vi "Roborealm image string.vi"(4 "remote port or service name":u16=1180, 6 "UP IP Address":string, 7 "Camera":string, 8 "error in (no error)":errorcluster, 9 "Width":string, 10 "Height":string, 11 "TCP Network Connection in":refnum<k5>) -> (0 "error out":errorcluster, 2 "connection ID out":refnum<k5>, 3 "String":string)   [LabVIEW 2017]
panel:
  out "img":string
  out "output 3":u32
  out "output 2":u32
  out "output 1":u32
  out "offset past scan":u32
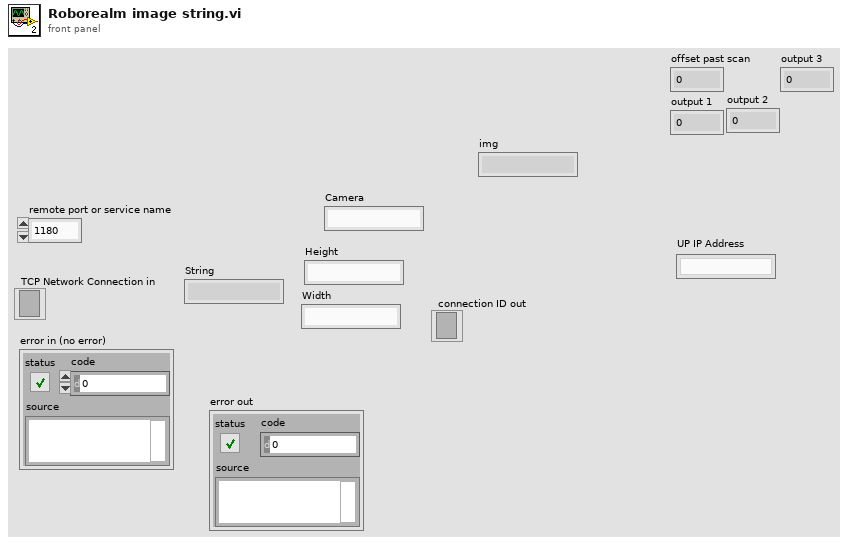
[diagram p1: front panel]
types:
  T1 = enum16{"Standard", "Buffered", "CRLF", "Immediate"}
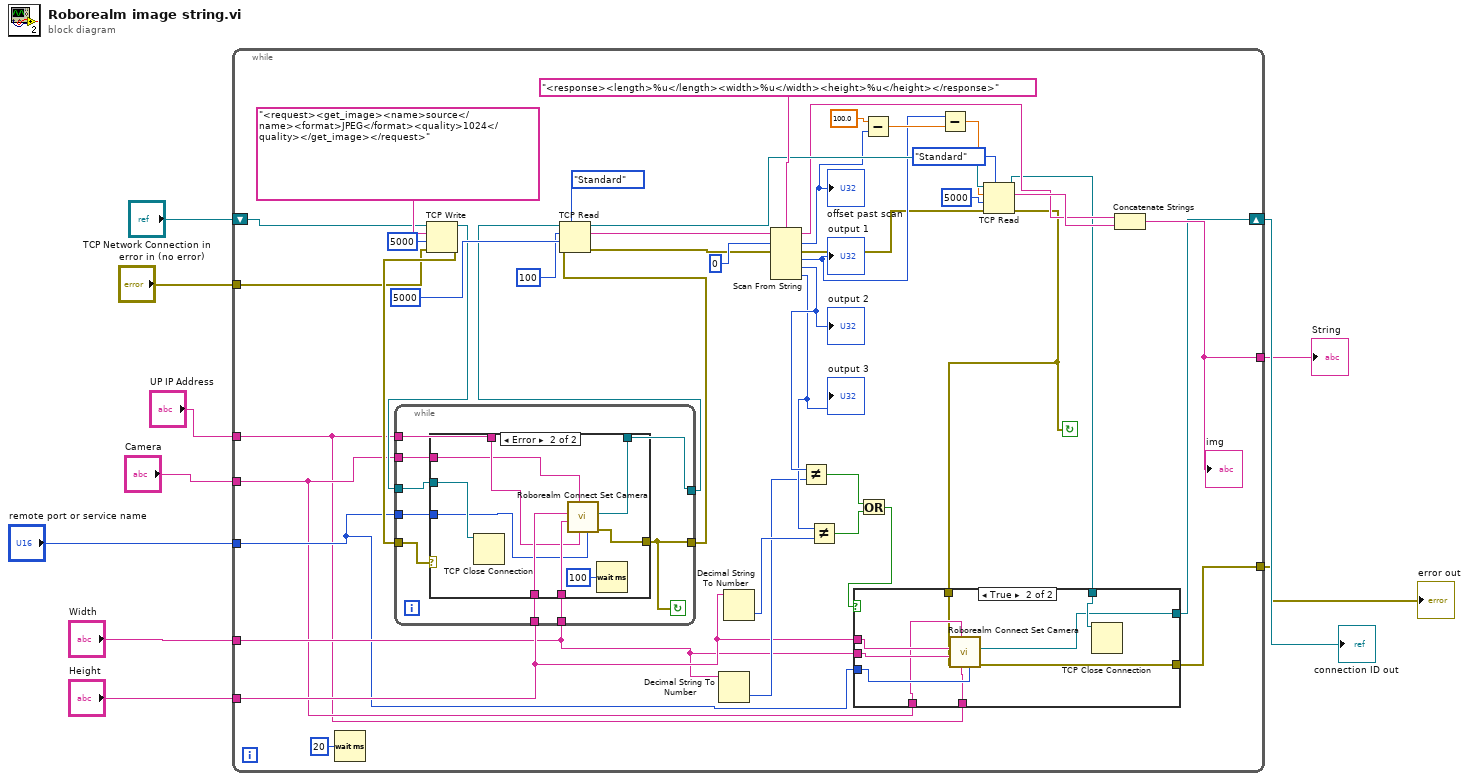
[diagram p0: block diagram]
diagram:
  n1 = while {
    tunnel: "UP IP Address" -> [w15]
    tunnel: [w33] -> w9
    tunnel: "remote port or service name" -> [w17]
    tunnel: "Width" -> [w18]
    tunnel: "Height" -> [w19]
    tunnel: "Camera" -> [w16]
    tunnel: [w12] -> w8
    shift-right: [w14] -> w10
    shift-left: "TCP Network Connection in" -> [w44]
    tunnel: "error in (no error)" -> [w11]
    stop <- w13 continue-if-true
    n2 = Wait (ms)(milliseconds to wait=u32 20) -> ()  [unwired: 1 out]
    n3 = TCP Write(connection ID=w44, data in="<request><get_image><name>source</name><format>JPEG</format><quality>1024</quality></get_image></request>", error in (no error)=w11, 9:5000 ("timeout ms (25000)")) -> (connection ID out=w36:refnum<k5>, error out=w46:errorcluster)  [unwired: 1 out]
    n4 = while {
      tunnel: w15 -> [w72]
      tunnel: [w71] -> w35
      tunnel: w36 -> [w70]
      tunnel: w46 -> [w74]
      tunnel: [w73] -> w45
      tunnel: w17 -> [w69]
      tunnel: w18 -> [w68]
      tunnel: w19 -> [w67]
      tunnel: w16 -> [w66]
      stop <- w73 continue-if-true
      n5 = case shown="Error" w74 {
        selector: w74 -> [w76 _]
        tunnel: [w76 w84] -> w73
        tunnel: [w75 w83] -> w71
        tunnel: w70 -> [w75 w82]
        tunnel: w72 -> [_ w79]
        tunnel: w69 -> [_ w78]
        tunnel: w68 -> [_ w81]
        tunnel: w67 -> [_ w80]
        tunnel: w66 -> [_ w77]
        frame No Error {
        }
        frame Error {
          n6 = TCP Close Connection(connection ID=w82) -> ()  [unwired: 2 in, 2 out]
          n7 = call "Roborealm Connect Set Camera.vi"("remote port or service name"=w78, "UP IP Address"=w79, "Camera"=w77, "Width"=w81, "Height"=w80) -> ("error out"=w84:errorcluster, "connection ID out"=w83:refnum<k5>)  [unwired: 5 in]
          n8 = Wait (ms)(milliseconds to wait=u32 100) -> ()  [unwired: 1 out]
        }
      }
    }
    n9 = TCP Read(connection ID=w35, bytes to read=100, error in (no error)=w45, 7:T1."Standard" ("mode (standard)"), 9:5000 ("bytes to read")) -> (connection ID out=w43:refnum<k5>, data out=w47:string, error out=w48:errorcluster)
    n10 = Decimal String To Number(string=w18) -> (number=w21:i32)  [unwired: 2 in, 1 out]
    n11 = Decimal String To Number(string=w19) -> (number=w26:i32)  [unwired: 2 in, 1 out]
    n12 = Scan From String(format string="<response><length>%u</length><width>%u</width><height>%u</height></response>", input string=w47, initial scan location=u32 0, error in=w48) -> (remaining string=w32:string, offset past scan=w37:u32, error out=w22:errorcluster, output 1=w30:u32, output 2=w28:u32, output 3=w27:u32)  [unwired: 3 in]
    "offset past scan" <- w37
    "output 1" <- w30
    "output 2" <- w28
    "output 3" <- w27
    n13 = Not Equal?(x=w28, y=w21) -> (x != y?=w25:bool)
    n14 = Not Equal?(x=w27, y=w26) -> (x != y?=w24:bool)
    n15 = Or(x=w25, y=w24) -> (x .or. y?=w23:bool)
    n16 = Subtract(x=100.0, y=w37) -> (x-y=w40:dbl)
    n17 = Subtract(x=w30, y=w40) -> (x-y=w39:dbl)
    n18 = TCP Read(connection ID=w43, bytes to read=w39, error in (no error)=w22, 7:T1."Standard" ("mode (standard)"), 9:5000 ("timeout ms (25000)")) -> (connection ID out=w20:refnum<k5>, data out=w34:string, error out=w13:errorcluster)
    n19 = case shown="True" w23 {
      tunnel: w20 -> [w56 w65]
      tunnel: w19 -> [_ w64]
      tunnel: w18 -> [_ w63]
      tunnel: w17 -> [_ w62]
      tunnel: w16 -> [_ w61]
      tunnel: w15 -> [_ w60]
      tunnel: [w55 w59] -> w12
      tunnel: [w56 w58] -> w14
      tunnel: w13 -> [w55 w57]
      frame False {
      }
      frame True {
        n20 = call "Roborealm Connect Set Camera.vi"("remote port or service name"=w62, "UP IP Address"=w60, "Camera"=w61, "error in (no error)"=w57, "Width"=w63, "Height"=w64) -> ("error out"=w59:errorcluster, "connection ID out"=w58:refnum<k5>)  [unwired: 4 in]
        n21 = TCP Close Connection(connection ID=w65) -> ()  [unwired: 2 in, 2 out]
      }
    }
    n22 = Concatenate Strings(w32, w34) -> (w33:string)
    "img" <- w33
  }
  "error out" <- w8
  "String" <- w9
  "connection ID out" <- w10
